vi "FunctionGraph.vi"() -> ()   [LabVIEW 2014]
uses:
  <vilib>/Analysis/1siggen.llb/Ramp Pattern by Samples.vi
  <vilib>/Analysis/NI_AALBase.lvlib
panel:
  in  "xmax":dbl=5.0
  in  "xmin":dbl=-5.0
  in  "Update":bool
  in  "stop":bool
  in  "w":dbl=1.0
  in  "A":dbl=1.0
  in  "Function":enum16{"A*sin(w*x)", "A*cos(w*x)", "A*tan(w*x)"}(ring)
  out "Function XY Graph":cluster{"Ramp Pattern":dbl[], dbl[]}(graph)
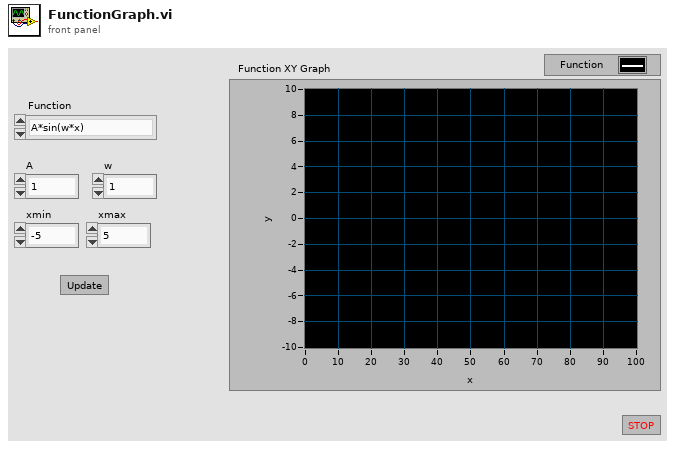
[diagram p1: front panel]
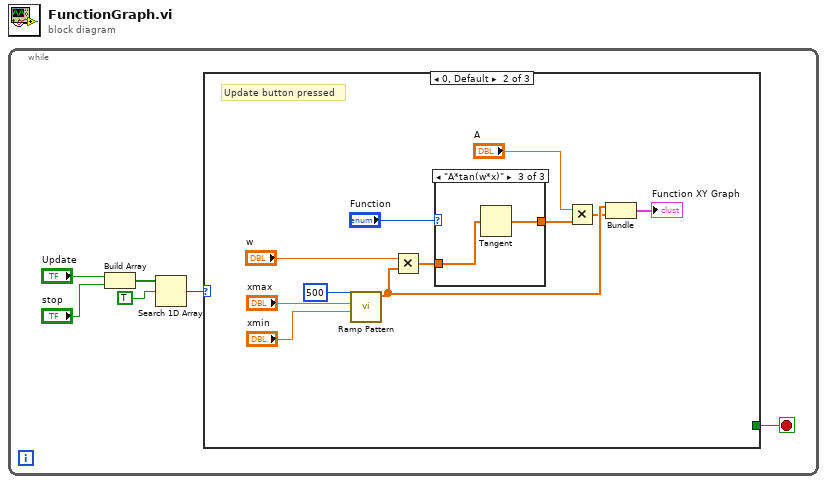
[diagram p0: block diagram]
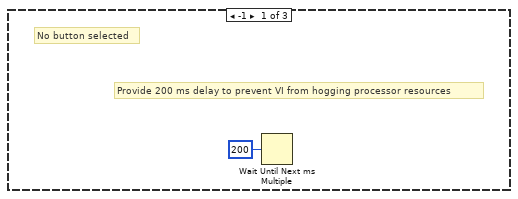
[diagram p2: hidden frame]
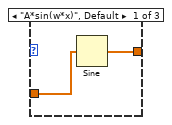
[diagram p3: hidden frame]
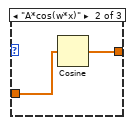
[diagram p4: hidden frame]
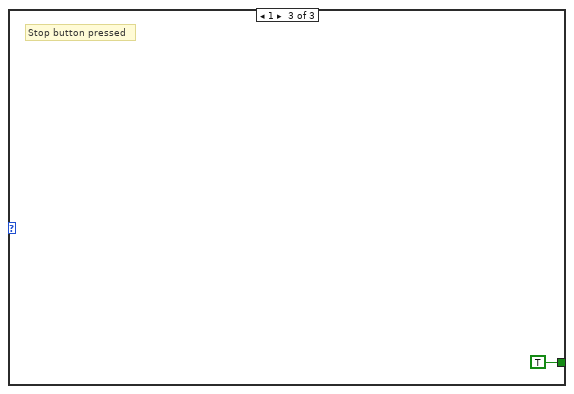
[diagram p5: hidden frame]
diagram:
  n1 = while {
    stop <- w1 stop-if-true
    n2 = Build Array("Update", "stop") -> (w4:bool[])
    n3 = Search 1D Array(1D array=w4, element=TRUE) -> (index of element=w2:i32)  [unwired: 1 in]
    n4 = case shown="0, Default" w2 {
      tunnel: [_ _ TRUE] -> w1
      frame -1 {
        # "Provide 200 ms delay to prevent VI from hogging processor resources"
        # "No button selected"
        n5 = Wait Until Next ms Multiple(millisecond multiple=u32 200) -> ()  [unwired: 1 out]
      }
      frame 0, Default {
        # "Update button pressed"
        n6 = call-poly <vilib>:"Ramp Pattern.vi"("start"="xmin", "end"="xmax", "samples"=500) -> ("Ramp Pattern"=w10:dbl[])  [unwired: 7 in, 1 out]
        n7 = Multiply(x="w", y=w10) -> (x*y=w13:dbl[])
        n8 = case shown="\"A*tan(w*x)\"" "Function" {
          tunnel: w13 -> [w20 w22 w24]
          tunnel: [w19 w21 w23] -> w12
          frame "A*sin(w*x)", Default {
            n9 = Sine(x=w20) -> (sin(x)=w19:dbl[])
          }
          frame "A*cos(w*x)" {
            n10 = Cosine(x=w22) -> (cos(x)=w21:dbl[])
          }
          frame "A*tan(w*x)" {
            n11 = Tangent(1:w24) -> (0:w23:dbl[])
          }
        }
        n12 = Multiply(x="A", y=w12) -> (x*y=w9:dbl[])
        n13 = Bundle("Ramp Pattern"=w10, w9) -> (→"Function XY Graph":cluster{"Ramp Pattern":dbl[], dbl[]})  [unwired: 1 in]
      }
      frame 1 {
        # "Stop button pressed"
      }
    }
  }
